vi "request auth code.vi"(8 "error in (no error)":errorcluster, 10 "Request URI":string, 11 "Oauth2 in":refnum<class "Oauth2.lvclass">) -> (0 "error out":errorcluster, 3 "Oauth2 out":refnum<class "Oauth2.lvclass">)   [LabVIEW 2017, in "Oauth2.lvclass"]
uses:
  Oauth2.lvclass
  <vilib>/Platform/browser.llb/Open URL in Default Browser (string).vi
panel:
  out "Response":string
  out "Header":string
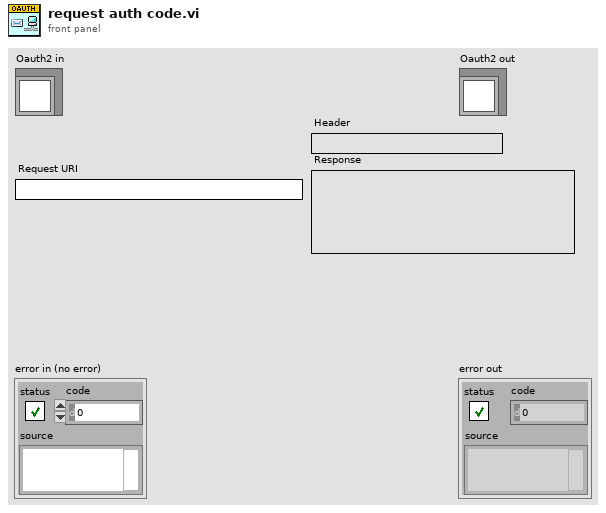
[diagram p1: front panel]
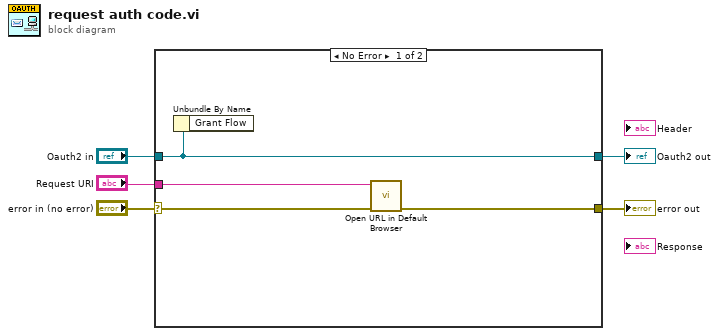
[diagram p0: block diagram]
diagram:
  n1 = case shown="No Error" "error in (no error)" {
    selector: "error in (no error)" -> [w8 w11]
    tunnel: [w7 w11] -> w4
    tunnel: [w6 w10] -> w2
    tunnel: "Oauth2 in" -> [w6 w10]
    tunnel: "Request URI" -> [w9 _]
    frame No Error {
      n2 = Unbundle By Name(w6) -> ()  [unwired: 1 out]
      n3 = call-poly <vilib>:"Open URL in Default Browser.vi"("error in (no error)"=w8, "URL"=w9) -> ("error out"=w7:errorcluster)  [unwired: 4 in, 1 out]
    }
    frame Error {
    }
  }
  "error out" <- w4
  "Oauth2 out" <- w2
